vi "TargetHeight.vi"() -> ()   [LabVIEW 2013]
panel:
  out "Height of target":dbl
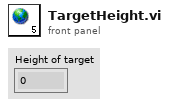
[diagram p1: front panel]
diagram:
